vi "ZuFaGen-1_V01.vi"(1 "Zeitlicher Abstand / ms":u32, 2 "Untre Grenze":dbl, 3 "Obere Grenze":dbl) -> (0 "Zufalszahl":dbl)   [LabVIEW 2022 SP3]
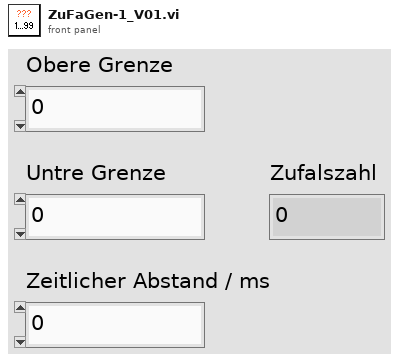
[diagram p1: front panel]
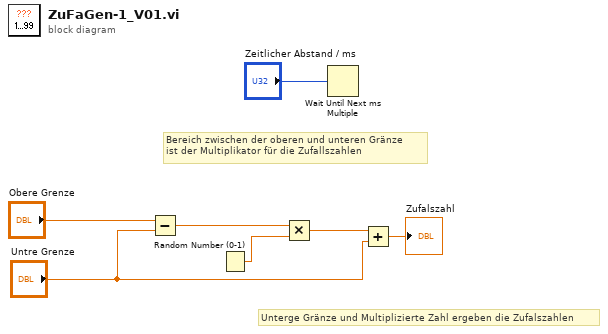
[diagram p0: block diagram]
diagram:
  # "Unterge Gränze und Multiplizierte Zahl ergeben die Zufalszahlen"
  # "Bereich zwischen der oberen und unteren Gränze \nist der Multiplikator für die Zufallszahlen"
  n1 = Subtract(x="Obere Grenze", y="Untre Grenze") -> (x-y=w5:dbl)
  n2 = Random Number (0-1)() -> (number: 0 to 1=w4:dbl)
  n3 = Multiply(x=w5, y=w4) -> (x*y=w3:dbl)
  n4 = Wait Until Next ms Multiple(millisecond multiple="Zeitlicher Abstand / ms") -> ()  [unwired: 1 out]
  n5 = Add(x=w3, y="Untre Grenze") -> (x+y=→"Zufalszahl":dbl)
